vi "okCFrontPanel Get Device Sensors.vi"(8 "Error In":errorcluster, 11 "okCFrontPanel Device Refnum":refnum<k24>) -> (0 "Error Out":errorcluster, 2 "Device Sensors Refnum":refnum<k24>, 3 "okCFrontPanel Device Refnum":refnum<k24>)   [LabVIEW 2021, in "okFrontPanelC#Wrapper.lvlib"]
uses:
  okFrontPanelC#Wrapper.lvlib
  D:/UCLA Thinkpad Google Drive/LabVIEW 2021 SP1/builds/SwissSPAD Live Distribution/Opal Kelly/C# Wrapper/v5.0.2/libFrontPanel-csharp.dll
  v5.0.2/libFrontPanel-csharp.dll
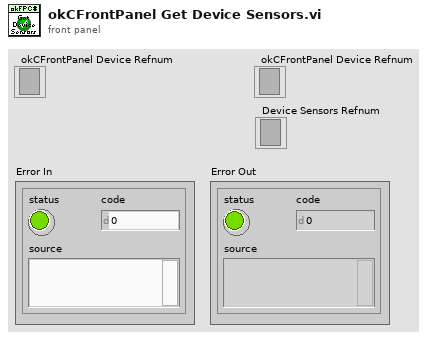
[diagram p1: front panel]
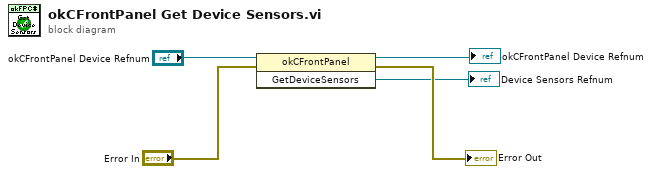
[diagram p0: block diagram]
diagram:
  n1 = invoke class="okCFrontPanel" method="GetDeviceSensors"(reference="okCFrontPanel Device Refnum", error in="Error In") -> (reference out=→"okCFrontPanel Device Refnum":refnum<k24>, error out=→"Error Out":errorcluster, "GetDeviceSensors"=→"Device Sensors Refnum":refnum<k24>)  [unwired: 1 in]
